vi "Actor Core.vi"(8 "error in":errorcluster, 11 "WebSocket Actor in":refnum<class "WebSocket Server.lvclass">) -> (0 "error out":errorcluster, 3 "Actor out":refnum<class "Actor.lvclass">)   [LabVIEW 2021, in "WebSocket Actors.lvlib" / "WebSocket Server.lvclass"]
doc: "(<B>Filename</B>: Actor Framework.lvlib:Actor.lvclass:Actor Core.vi)\n\nReceives messages to the actor, reacts to them, and initiates any error handling that may shut the actor down.\n\nDescendant classes may override this VI to append parallel tasks for the actor to complete while it handles messages. Overrides use the Call Parent Method node."
uses:
  WebSocket Server.lvclass
  C:/Program Files/National Instruments/LabVIEW 2021/vi.lib/ActorFramework/Actor/Actor.lvclass
  <vilib>/ActorFramework/Actor/Actor.lvclass
  <vilib>/ActorFramework/Actor/Actor.lvclass/Actor.ctl
  <vilib>/ActorFramework/Message Enqueuer/Message Enqueuer.lvclass/Message Enqueuer.ctl
  WebSocket Server.lvclass/WebSocket Server.ctl
  <vilib>/ActorFramework/Report Error Msg/Report Error Msg.lvclass/Report Error Msg.ctl
  <vilib>/GPower/Error/Library/Filter/FilterSingle.vi
  <vilib>/ActorFramework/Message Enqueuer/Init from Existing Queue.vi
  <vilib>/GPower/Error/Library/SplitAppended.vi
  <vilib>/ActorFramework/Message Enqueuer/Enqueue.vi
  <vilib>/GPower/Error/Library/SubVIs/ExplanationToError.vi
  <vilib>/dlg_ctls.llb/Space Constant.vi
  <vilib>/ActorFramework/Report Error Msg/Report Error Msg.lvclass
  C:/Program Files/National Instruments/LabVIEW 2021/vi.lib/ActorFramework/Message/Message.lvclass
  <vilib>/ActorFramework/Stop Msg/Stop Msg.lvclass
  <vilib>/Utility/error.llb/Error Cluster From Error Code.vi
  <vilib>/Utility/error.llb/Trim Whitespace.vi
  <vilib>/Utility/error.llb/Error Code Database.vi
  <vilib>/GPower/Error/Library/Append/AppendSingle.vi
  <vilib>/Utility/LVClass/Get LV Class Name.vi
  <resource>/AFDebug/Generate Trace for Message.vi
  <vilib>/ActorFramework/Message Priority Queue/Priority Enqueue.vi
  <vilib>/ActorFramework/Message Enqueuer/Message Enqueuer.lvclass
  <vilib>/ErrorRing/Error Ring.xnode
  WebSocket Server Messages/Write listener ID Msg/Write listener ID Msg.lvclass
  WebSocket Server Messages/Add Client to Service Msg/Add Client to Service Msg.lvclass
  <vilib>/GPower/Error/GPError.lvlib
  <userlib>/_OpenG.lib/error/error.llb/openg_error.lvlib
  C:/Projects/WebSocket-Actor/WebSocket Actor/WebSocket Server/WebSocket Server.lvclass
  WebSocket Server Messages/Write Listener Down Msg/Write Listener Down Msg.lvclass
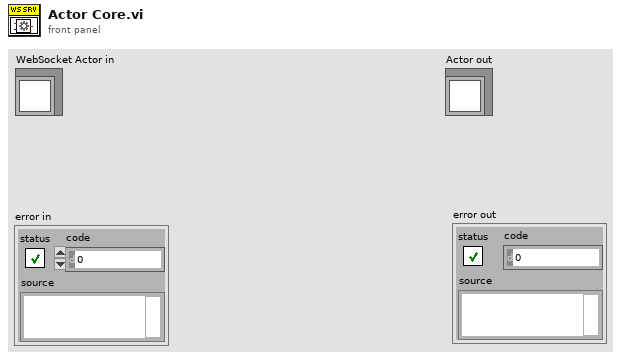
[diagram p1: front panel]
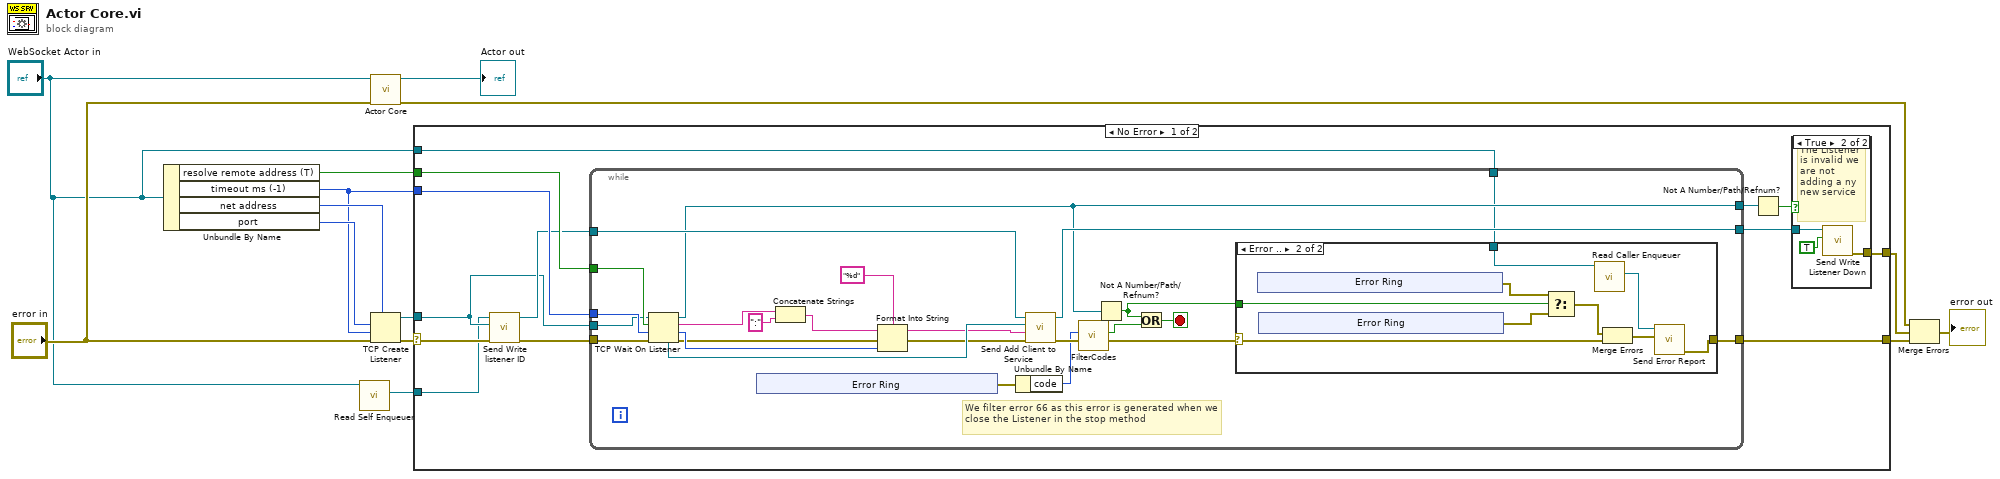
[diagram p0: block diagram]
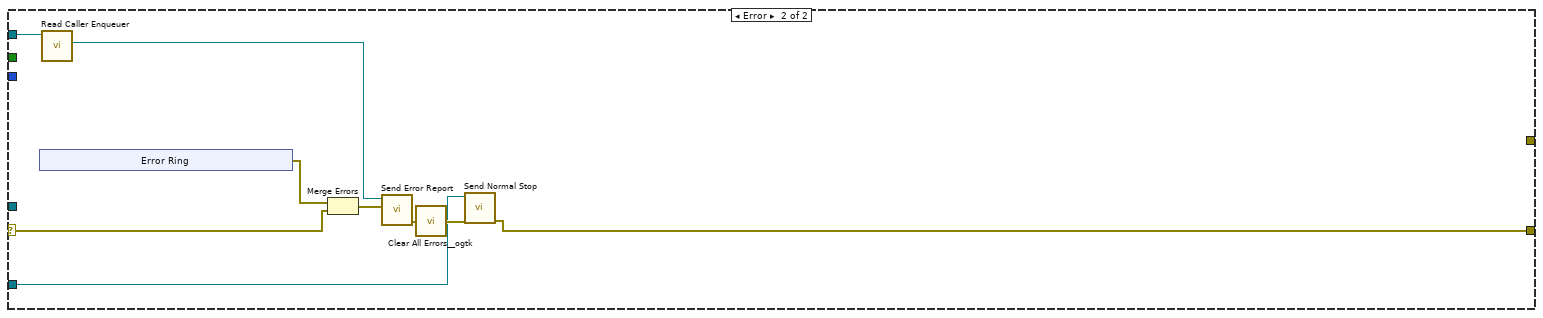
[diagram p4: hidden frame]
diagram:
  n1 = Unbundle By Name("WebSocket Actor in") -> ("resolve remote address (T)"=w12:bool, "timeout ms (-1)"=w8:i32, "net address"=w9:u32, "port"=w10:u16)
  n2 = call <vilib>:"Read Self Enqueuer.vi"("Actor"="WebSocket Actor in") -> ("Self Enqueuer"=w3:refnum<class "Message Enqueuer.lvclass">)  [unwired: 10 in]
  n3 = call-parent "Actor Core.vi"("error in"="error in", "Actor in"="WebSocket Actor in") -> ("error out"=w14:errorcluster, "Actor out"=→"Actor out":refnum<class "Actor.lvclass">)  [unwired: 8 in]
  n4 = TCP Create Listener(7:w9, 8:"error in", 9:w8, 10:w10) -> (0:w7:errorcluster, 3:w6:refnum<k5>)  [unwired: 1 in, 1 out]
  n5 = case shown="No Error" w7 {
    selector: w7 -> [w25 w85]
    tunnel: w12 -> [w27 _]
    tunnel: w8 -> [w26 _]
    tunnel: w6 -> [w22 _]
    tunnel: [w21 w78] -> w4
    tunnel: w3 -> [w20 w79]
    tunnel: "WebSocket Actor in" -> [w19 w80]
    tunnel: [w15 _] -> w1
    frame No Error {
      n6 = call "Send Write listener ID.vi"("error in (no error)"=w25, "listener ID"=w22, "Message Enqueuer in"=w20) -> ("error out"=w23:errorcluster, "Message Enqueuer out"=w24:refnum<class "Message Enqueuer.lvclass">)  [unwired: 7 in]
      n7 = while {
        tunnel: w27 -> [w50]
        tunnel: w26 -> [w52]
        tunnel: w24 -> [w49]
        tunnel: w23 -> [w48]
        tunnel: w22 -> [w47]
        tunnel: [w32] -> w21
        tunnel: [w36] -> w18
        tunnel: [w37] -> w17
        tunnel: w19 -> [w33]
        stop <- w38 stop-if-true
        # "We filter error 66 as this error is generated when we close the Listener in the stop method"
        n8 = TCP Wait On Listener(8:w48, 9:w52, 10:w50, 11:w47) -> (0:w42:errorcluster, 1:w45:u16, 2:w46:string, 3:w36:refnum<k5>, 4:w51:refnum<k5>)
        n9 = xnode "Error Ring"() -> ("error out"=w55:errorcluster)
        n10 = Concatenate Strings(w46, ":" ("string")) -> (w43:string)
        n11 = Format Into String(format string="%d", initial string=w43, error in=w42, w45) -> (resulting string=w40:string, error out=w41:errorcluster)
        n12 = Unbundle By Name(w55) -> ("code"=w53:i32)
        n13 = call "Send Add Client to Service.vi"("error in (no error)"=w41, "Client ID"=w40, "WebSocket Connection in"=w51, "Message Enqueuer in"=w49) -> ("error out"=w54:errorcluster, "Message Enqueuer out"=w37:refnum<class "Message Enqueuer.lvclass">)  [unwired: 6 in]
        n14 = call-poly <vilib>:"FilterCodes.vi"("Error in"=w54, "Code to filter"=w53) -> ("Error out"=w34:errorcluster, "Code filtered?"=w35:bool)  [unwired: 8 in]
        n15 = Not A Number/Path/Refnum?(number/path/refnum=w36) -> (NaN/Path/Refnum?=w31:bool)
        n16 = Or(x=w31, y=w35) -> (x .or. y?=w38:bool)
        n17 = case shown="Error .." w34 {
          selector: w34 -> [w56 w64]
          tunnel: w33 -> [_ w63]
          tunnel: [w56 w61] -> w32
          tunnel: w31 -> [_ w58]
          frame No Error {
          }
          frame Error {
            n18 = xnode "Error Ring"() -> ("error out"=w59:errorcluster)
            n19 = xnode "Error Ring"() -> ("error out"=w60:errorcluster)
            n20 = Select(t=w59, s=w58, f=w60) -> (s? t:f=w57:errorcluster)
            n21 = call <vilib>:"Read Caller Enqueuer.vi"("Actor"=w63) -> ("Caller Enqueuer"=w62:refnum<class "Message Enqueuer.lvclass">)  [unwired: 10 in]
            n22 = Merge Errors(w57, w64) -> (w65:errorcluster)
            n23 = call <vilib>:"Send Error Report.vi"("Error From Sender"=w65, "Message Enqueuer"=w62) -> ("error out"=w61:errorcluster)  [unwired: 9 in]
          }
        }
      }
      n24 = Not A Number/Path/Refnum?(number/path/refnum=w18) -> (NaN/Path/Refnum?=w16:bool)
      n25 = case shown="True" w16 {
        tunnel: w17 -> [_ w30]
        tunnel: [_ w29] -> w15
        frame False {
        }
        frame True {
          # "The Listener is invalid we are not adding a ny new service"
          n26 = call "Send Write Listener Down.vi"("Listener Down"=TRUE, "Message Enqueuer in"=w30) -> ("error out"=w29:errorcluster)  [unwired: 8 in, 1 out]
        }
      }
    }
    frame Error {
      n27 = xnode "Error Ring"() -> ("error out"=w86:errorcluster)
      n28 = call <vilib>:"Read Caller Enqueuer.vi"("Actor"=w80) -> ("Caller Enqueuer"=w83:refnum<class "Message Enqueuer.lvclass">)  [unwired: 10 in]
      n29 = Merge Errors(w86, w85) -> (w84:errorcluster)
      n30 = call <vilib>:"Send Error Report.vi"("Error From Sender"=w84, "Message Enqueuer"=w83) -> ("error out"=w82:errorcluster)  [unwired: 9 in]
      n31 = call <userlib>:"Clear All Errors__ogtk.vi"("Error In"=w82) -> ("Error Out"=w81:errorcluster)  [unwired: 3 in]
      n32 = call <vilib>:"Send Normal Stop.vi"("error in (no error)"=w81, "Message Enqueuer"=w79) -> ("error out"=w78:errorcluster)  [unwired: 9 in]
    }
  }
  n33 = Merge Errors(w14, w1, w4) -> (→"error out":errorcluster)
